vi "Read SA Pin.vi"(8 "error in (no error)":errorcluster, 11 "LTE_ModAcc in":refnum<class "LTE_ModAcc.lvclass">=refnum) -> (0 "error out":errorcluster, 2 "SA Pin":string, 3 "LTE_ModAcc out":refnum<class "LTE_ModAcc.lvclass">)   [LabVIEW 2016, in "SeqAuto Evaluations.lvlib" / "LTE_ModAcc.lvclass"]
uses:
  LTE_ModAcc.lvclass
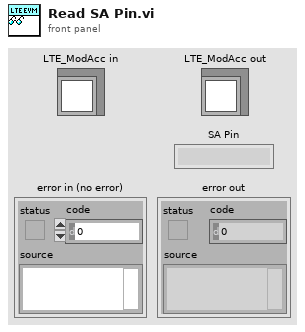
[diagram p1: front panel]
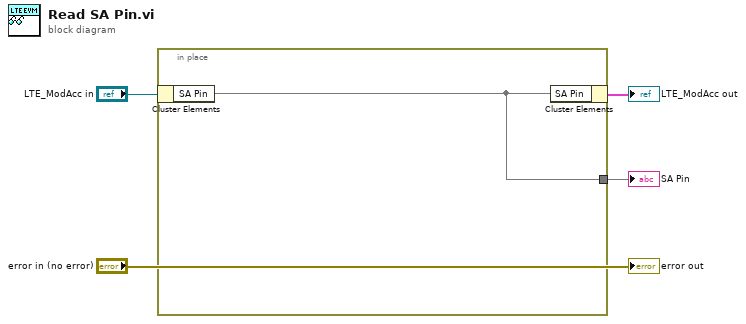
[diagram p0: block diagram]
diagram:
  n1 = in-place {
    in-place-border: [w5] -> w1
    n2 = in-place-cluster #1("LTE_ModAcc in") -> ("SA Pin"=w5)
    n3 = in-place-cluster #1("SA Pin"=w5) -> (→"LTE_ModAcc out":cluster{})
  }
  "SA Pin" <- w1
  "error out" <- "error in (no error)"
